vi "Image Subtract.vi"(5 "Image Height":u16=512, 6 "Enable DRAM":bool, 7 "Image Width":u16=512, 8 "Pixel Valid":bool, 11 "Pixel Data":u64) -> (0 "Output Valid?":bool, 3 "Pixel Data":u64, 4 "Pixel Mask":u64)   [LabVIEW 2015]
uses:
  Controls (FPGA)/DRAM Data.ctl
  <vilib>/rvi/DataTransferAndStorage/Container/Common/niFpgaContainerGetUniqueNameForEmu.vi
  <vilib>/rvi/DataTransferAndStorage/Container/Common/niFpgaContainerSetEmuInfo.vi
  <vilib>/rvi/eio/common/nirviEmuReportErrorAndStop.vi
  <vilib>/rvi/Emulation/niFpgaEmulationIsFPGAContextNoSignature.vi
  <vilib>/rvi/Emulation/niFpgaSctlEmulationGetInTimedLoop.vi
  <vilib>/rvi/errors/niFpgaSetErrorForExecOnDevCompSimple.vi
  <vilib>/rvi/FIFO/Fifo_Resource/nirvififoEmulationSetSize.vi
  <vilib>/rvi/FIFO/Fifo_Resource/nirviFifoEmulationQueueMgr.vi
  <instcachedir>/0/nirviFifoEmulationQueueMgr_E5CAEC123FF24DC58D834DCA3CDAA9B5.lvgen/nirviFifoEmulationQueueMgr_E5CAEC123FF24DC58D834DCA3CDAA9B5_006.vi
  <vilib>/Utility/error.llb/Clear Errors.vi
  <vilib>/rvi/FIFO/Fifo_Resource/nirvififoEmulationCreateLock.vi
  <vilib>/rvi/Emulation/niFpgaProcessEmulError.vi
  <vilib>/rvi/FIFO/Fifo_Resource/nirvififoEmulationObtainLock.vi
  <vilib>/rvi/FIFO/Fifo_Resource/nirvififoEmulationReleaseLock.vi
  <vilib>/rvi/occurrence/nirviWaitOnOccurrenceBase.vi
  <vilib>/rvi/errors/nirviReportUnexpectedCaseInternalError.vi
  <vilib>/rvi/errors/nirviReportUnexpectedCaseInternalError (U32).vi
  <vilib>/rvi/FIFO/Fifo_Resource/nirvififoEmulationDetermineInputValidOut.vi
  <vilib>/rvi/eio/common/nirviEmuTemplateMethod_errors.vi
  <vilib>/rvi/LocalResourceManager/LocalResourceManager.xnode
  <vilib>/rvi/DataTransferAndStorage/Container/XNode/niFpgaContainer.xnode
  <vilib>/rvi/FIFO/Fifo_Resource/nirvififoEmulationRead.vi
  <vilib>/rvi/FIFO/Fifo_Resource/nirvififoEmulationWrite.vi
  <vilib>/eio/EIONode/EIONode.xnode
  <vilib>/rvi/FIFO/Fifo_Resource/nirvififoEmulationGetNumberOfElementsToWrite.vi
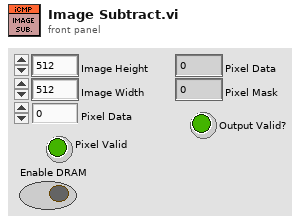
[diagram p1: front panel]
types:
  T1 = typedef "DRAM Data.ctl" = cluster{"Lower 64":u64, "Upper 64":u64}
  T2 = cluster{"Numeric Control":u8, "Numeric Control":u8, "Numeric Control":u8, "Numeric Control":u8, "Numeric Control":u8, "Numeric Control":u8, "Numeric Control":u8, "Numeric Control":u8}
  T3 = cluster{"Numeric Control":i16, "Numeric Control":i16, "Numeric Control":i16, "Numeric Control":i16, "Numeric Control":i16, "Numeric Control":i16, "Numeric Control":i16, "Numeric Control":i16}
  T4 = cluster{"Numeric Control":bool, "Numeric Control":bool, "Numeric Control":bool, "Numeric Control":bool, "Numeric Control":bool, "Numeric Control":bool, "Numeric Control":bool, "Numeric Control":bool}
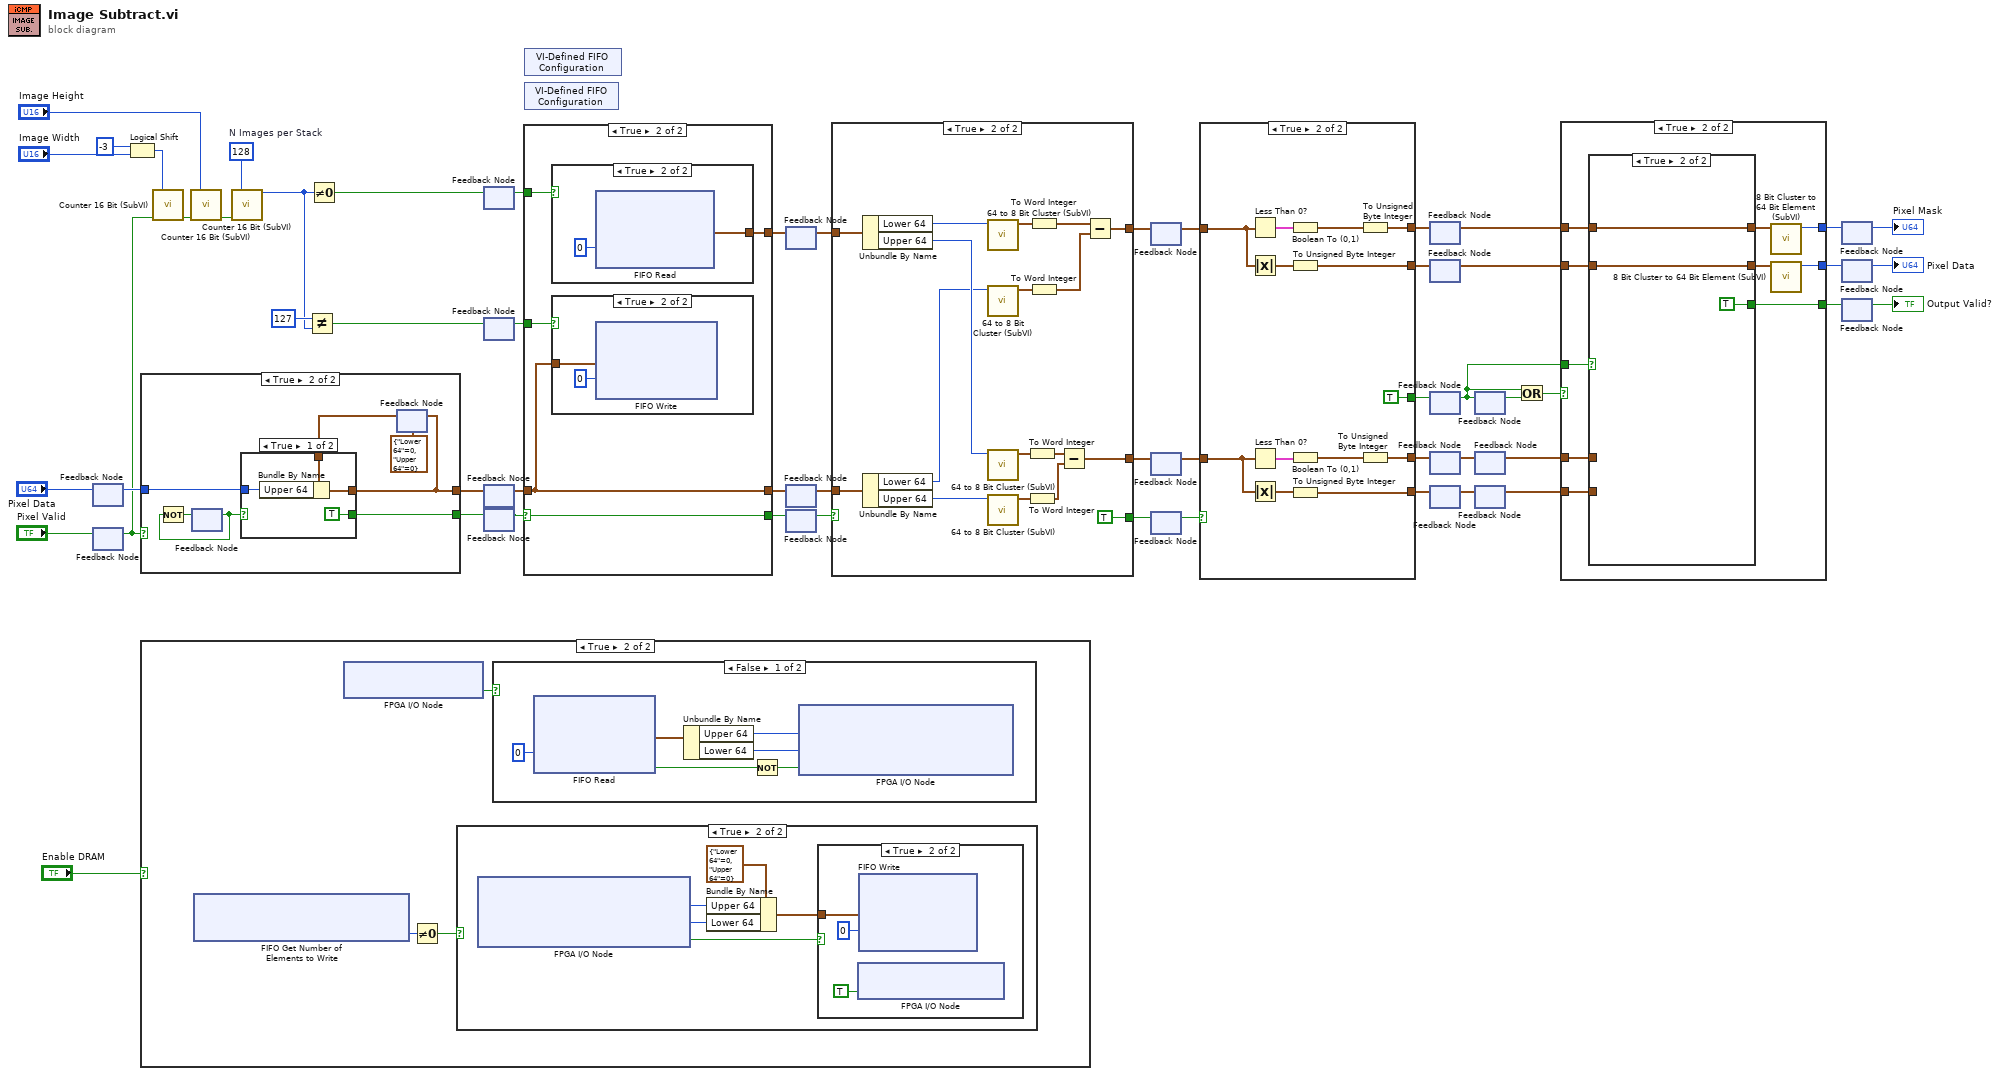
[diagram p0: block diagram]
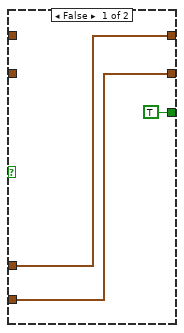
[diagram p7: hidden frame]
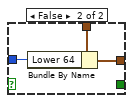
[diagram p14: hidden frame]
diagram:
  w43 = u16 128  # N Images per Stack
  n1 = feedback-in #1("Pixel Data") -> ()
  n2 = feedback #1() -> (w50:u64)  [unwired: 1 in]
  n3 = feedback-in #2("Pixel Valid") -> ()
  n4 = feedback #2() -> (w48:bool)  [unwired: 1 in]
  n5 = Logical Shift(y=i16 -3, x="Image Width") -> (x << y=w2:u16)
  n6 = case shown="True" w48 {
    tunnel: w50 -> [_ w59]
    tunnel: [_ w56] -> w52
    tunnel: [_ w55] -> w51
    frame False {
    }
    frame True {
      n7 = feedback #3() -> (w58:bool)  [unwired: 1 in]
      n8 = Not(x=w58) -> (.not. x?=w57:bool)
      n9 = feedback-in #3(w57) -> ()
      n10 = feedback #4(T1 {"Lower 64"=0, "Upper 64"=0}) -> (w60:T1)
      n11 = case shown="True" w58 {
        tunnel: [w65 w68] -> w56
        tunnel: w60 -> [w64 w67]
        tunnel: w59 -> [w63 w66]
        tunnel: [TRUE _] -> w55
        frame True {
          n12 = Bundle By Name(cluster=w64, "Upper 64"=w63) -> (w65:T1)
        }
        frame False {
          n13 = Bundle By Name(cluster=w67, "Lower 64"=w66) -> (w68:T1)
        }
      }
      n14 = feedback-in #4(w56) -> ()
    }
  }
  n15 = case shown="True" "Enable DRAM" {
    frame False {
    }
    frame True {
      n16 = xnode ("FIFO Get Number of Elements to Write")() -> ("Number of Elements to Write"=w70:u32)  [unwired: 1 in, 1 out]
      n17 = xnode "FPGA I/O Node"() -> ("DRAM Bank 0\\Full"=w71:bool)  [unwired: 1 in, 1 out]
      n18 = Not Equal To 0?(x=w70) -> (x != 0?=w69:bool)
      n19 = case shown="True" w69 {
        frame False {
        }
        frame True {
          n20 = xnode "FPGA I/O Node"() -> ("DRAM Bank 0\\Read_Data_Upper"=w76:u64, "DRAM Bank 0\\Read_Data_Lower"=w75:u64, "DRAM Bank 0\\Data_Available"=w72:bool)  [unwired: 3 in, 3 out]
          n21 = Bundle By Name(cluster=T1 {"Lower 64"=0, "Upper 64"=0}, "Upper 64"=w76, "Lower 64"=w75) -> (w73:T1)
          n22 = case shown="True" w72 {
            tunnel: w73 -> [_ w79]
            frame False {
            }
            frame True {
              n23 = xnode "FPGA I/O Node"("DRAM Bank 0\\Read"=TRUE ("DRAM Bank 0\\Read")) -> ()  [unwired: 1 in, 1 out]
              n24 = xnode ("FIFO Write")("Element"=w79, "Timeout"=0) -> ()  [unwired: 1 in, 2 out]
            }
          }
        }
      }
      n25 = case shown="False" w71 {
        frame False {
          n26 = xnode ("FIFO Read")("Timeout"=0) -> ("Element"=w82:cluster{"Lower 64":u64, "Upper 64":u64}, "Timed Out?"=w84:bool)  [unwired: 1 in, 1 out]
          n27 = Unbundle By Name(w82) -> ("Upper 64"=w80:u64, "Lower 64"=w81:u64)
          n28 = Not(x=w84) -> (.not. x?=w83:bool)
          n29 = xnode "FPGA I/O Node"("DRAM Bank 0\\Write_Data_Upper"=w80, "DRAM Bank 0\\Write_Data_Lower"=w81, "DRAM Bank 0\\Write"=w83) -> ()  [unwired: 3 in, 3 out]
        }
        frame True {
        }
      }
    }
  }
  n30 = call "Counter 16 Bit (SubVI).vi"("Max. Count"=w2, "Enable"=w48) -> ("Count End?"=w45:bool)  [unwired: 11 in, 2 out]
  n31 = call "Counter 16 Bit (SubVI).vi"("Max. Count"="Image Height", "Enable"=w45) -> ("Count End?"=w44:bool)  [unwired: 11 in, 2 out]
  n32 = call "Counter 16 Bit (SubVI).vi"("Max. Count"=w43, "Enable"=w44) -> ("Count"=w40:u16)  [unwired: 11 in, 2 out]
  n33 = Not Equal?(x=u16 127, y=w40) -> (x != y?=w41:bool)
  n34 = Not Equal To 0?(x=w40) -> (x != 0?=w37:bool)
  n35 = feedback-in #5(w37) -> ()
  n36 = feedback #5() -> (w36:bool)  [unwired: 1 in]
  n37 = feedback-in #6(w41) -> ()
  n38 = feedback #6() -> (w38:bool)  [unwired: 1 in]
  n39 = feedback-in #7(w52) -> ()
  n40 = feedback #7() -> (w49:T1)  [unwired: 1 in]
  n41 = feedback-in #8(w51) -> ()
  n42 = feedback #8() -> (w39:bool)  [unwired: 1 in]
  n43 = case shown="True" w39 {
    selector: w39 -> [_ w87]
    tunnel: w49 -> [_ w88]
    tunnel: w38 -> [_ w90]
    tunnel: w36 -> [_ w89]
    tunnel: [_ w88] -> w35
    tunnel: [_ w87] -> w31
    tunnel: [_ w86] -> w34
    frame False {
    }
    frame True {
      n44 = case shown="True" w89 {
        tunnel: [_ w91] -> w86
        frame False {
        }
        frame True {
          n45 = xnode ("FIFO Read")("Timeout"=0) -> ("Element"=w91:cluster{"Lower 64":u64, "Upper 64":u64})  [unwired: 1 in, 2 out]
        }
      }
      n46 = case shown="True" w90 {
        tunnel: w88 -> [_ w94]
        frame False {
        }
        frame True {
          n47 = xnode ("FIFO Write")("Element"=w94, "Timeout"=0) -> ()  [unwired: 1 in, 2 out]
        }
      }
    }
  }
  n48 = xnode "VI-Defined FIFO Configuration"() -> ()  [unwired: 1 out]
  n49 = xnode "VI-Defined FIFO Configuration"() -> ()  [unwired: 1 out]
  n50 = feedback-in #9(w34) -> ()
  n51 = feedback #9() -> (w30:cluster{"Lower 64":u64, "Upper 64":u64})  [unwired: 1 in]
  n52 = feedback-in #10(w35) -> ()
  n53 = feedback #10() -> (w29:T1)  [unwired: 1 in]
  n54 = feedback-in #11(w31) -> ()
  n55 = feedback #11() -> (w28:bool)  [unwired: 1 in]
  n56 = case shown="True" w28 {
    tunnel: w29 -> [_ w111]
    tunnel: w30 -> [_ w110]
    tunnel: [_ w97] -> w33
    tunnel: [_ w96] -> w32
    tunnel: [_ TRUE] -> w27
    frame False {
    }
    frame True {
      n57 = Unbundle By Name(w110) -> ("Lower 64"=w109:u64, "Upper 64"=w108:u64)
      n58 = Unbundle By Name(w111) -> ("Lower 64"=w106:u64, "Upper 64"=w107:u64)
      n59 = call "64 to 8 Bit Cluster (SubVI).vi"("Data In"=w109) -> ("Data Out"=w105:T2)  [unwired: 10 in]
      n60 = call "64 to 8 Bit Cluster (SubVI).vi"("Data In"=w106) -> ("Data Out"=w104:T2)  [unwired: 10 in]
      n61 = call "64 to 8 Bit Cluster (SubVI).vi"("Data In"=w108) -> ("Data Out"=w101:T2)  [unwired: 10 in]
      n62 = call "64 to 8 Bit Cluster (SubVI).vi"("Data In"=w107) -> ("Data Out"=w100:T2)  [unwired: 10 in]
      n63 = To Word Integer(number=w101) -> (16bit integer=w99:T3)
      n64 = To Word Integer(number=w100) -> (16bit integer=w98:T3)
      n65 = To Word Integer(number=w105) -> (16bit integer=w103:T3)
      n66 = To Word Integer(number=w104) -> (16bit integer=w102:T3)
      n67 = Subtract(x=w99, y=w98) -> (x-y=w96:T3)
      n68 = Subtract(x=w103, y=w102) -> (x-y=w97:T3)
    }
  }
  n69 = feedback-in #12(w33) -> ()
  n70 = feedback #12() -> (w26:T3)  [unwired: 1 in]
  n71 = feedback-in #13(w32) -> ()
  n72 = feedback #13() -> (w25:T3)  [unwired: 1 in]
  n73 = feedback-in #14(w27) -> ()
  n74 = feedback #14() -> (w24:bool)  [unwired: 1 in]
  n75 = case shown="True" w24 {
    tunnel: w26 -> [_ w124]
    tunnel: w25 -> [_ w123]
    tunnel: [_ w118] -> w14
    tunnel: [_ w117] -> w18
    tunnel: [_ w116] -> w15
    tunnel: [_ w115] -> w19
    tunnel: [_ TRUE] -> w23
    frame False {
    }
    frame True {
      n76 = Less Than 0?(x=w124) -> (x < 0?=w122:T4)
      n77 = Absolute Value(x=w124) -> (abs(x)=w120:T3)
      n78 = Less Than 0?(x=w123) -> (x < 0?=w121:T4)
      n79 = Absolute Value(x=w123) -> (abs(x)=w119:T3)
      n80 = Boolean To (0,1)(Boolean=w122) -> (0, 1=w113:T3)
      n81 = To Unsigned Byte Integer(number=w120) -> (unsigned 8bit integer=w115:T2)
      n82 = Boolean To (0,1)(Boolean=w121) -> (0, 1=w112:T3)
      n83 = To Unsigned Byte Integer(number=w119) -> (unsigned 8bit integer=w117:T2)
      n84 = To Unsigned Byte Integer(number=w113) -> (unsigned 8bit integer=w116:T2)
      n85 = To Unsigned Byte Integer(number=w112) -> (unsigned 8bit integer=w118:T2)
    }
  }
  n86 = feedback-in #15(w15) -> ()
  n87 = feedback #15() -> (w13:T2)  [unwired: 1 in]
  n88 = feedback-in #16(w19) -> ()
  n89 = feedback #16() -> (w16:T2)  [unwired: 1 in]
  n90 = feedback #17() -> (w20:bool)  [unwired: 1 in]
  n91 = feedback-in #17(w23) -> ()
  n92 = feedback-in #18(w14) -> ()
  n93 = feedback #18() -> (w12:T2)  [unwired: 1 in]
  n94 = feedback-in #19(w18) -> ()
  n95 = feedback #19() -> (w17:T2)  [unwired: 1 in]
  n96 = feedback #20() -> (w21:bool)  [unwired: 1 in]
  n97 = feedback-in #20(w20) -> ()
  n98 = feedback-in #21(w12) -> ()
  n99 = feedback #21() -> (w11:T2)  [unwired: 1 in]
  n100 = feedback-in #22(w17) -> ()
  n101 = feedback #22() -> (w10:T2)  [unwired: 1 in]
  n102 = Or(x=w20, y=w21) -> (x .or. y?=w22:bool)
  n103 = case shown="True" w22 {
    tunnel: w20 -> [_ w134]
    tunnel: w16 -> [_ w133]
    tunnel: [_ w132] -> w8
    tunnel: w10 -> [_ w131]
    tunnel: w13 -> [_ w130]
    tunnel: w11 -> [_ w129]
    tunnel: [_ w125] -> w7
    tunnel: [_ w126] -> w9
    frame False {
    }
    frame True {
      n104 = case shown="True" w134 {
        tunnel: w133 -> [_ w140]
        tunnel: [w136 w140] -> w127
        tunnel: [TRUE TRUE] -> w132
        tunnel: w131 -> [w136 _]
        tunnel: w130 -> [_ w138]
        tunnel: w129 -> [w135 _]
        tunnel: [w135 w138] -> w128
        frame False {
        }
        frame True {
        }
      }
      n105 = call "8 Bit Cluster to 64 Bit Element (SubVI).vi"("Pixel Cluster"=w128) -> ("Pixel Data (64-Bit)"=w125:u64)  [unwired: 10 in]
      n106 = call "8 Bit Cluster to 64 Bit Element (SubVI).vi"("Pixel Cluster"=w127) -> ("Pixel Data (64-Bit)"=w126:u64)  [unwired: 10 in]
    }
  }
  n107 = feedback-in #23(w7) -> ()
  n108 = feedback #23() -> (→"Pixel Mask":u64)  [unwired: 1 in]
  n109 = feedback-in #24(w9) -> ()
  n110 = feedback #24() -> (→"Pixel Data":u64)  [unwired: 1 in]
  n111 = feedback-in #25(w8) -> ()
  n112 = feedback #25() -> (→"Output Valid?":bool)  [unwired: 1 in]
